vi "解析数据.vi"(8 "error in (no error)":errorcluster caption="错误输入（无错误）", 9 "当前模块数据属性":T1(array[cluster]), 10 "当前模块上一次的值":string[](array[string]), 11 "配置信息":string[](array[string])) -> (0 "error out":errorcluster caption="错误输出", 3 "输出数据":string)   [LabVIEW 2014]
doc: "该模板用于创建子VI。"
uses:
  glb/glb_data.vi
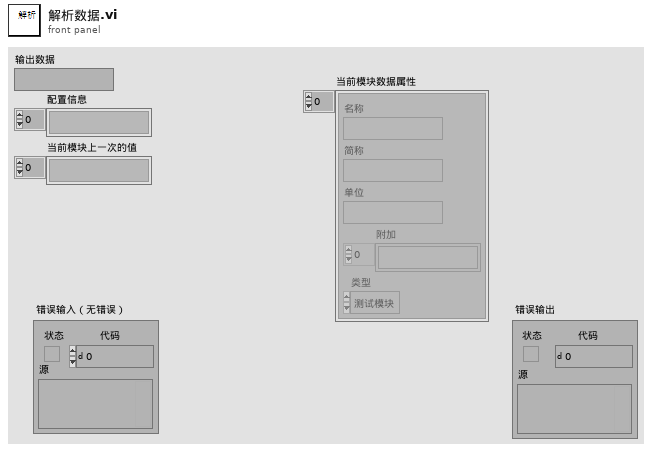
[diagram p1: front panel]
types:
  T1 = cluster{"名称":string, "简称":string, "单位":string, "附加":string[], "类型":enum16{"测试模块", "FPGA", "cRIO", "其他设备", "总体展示"}}[]
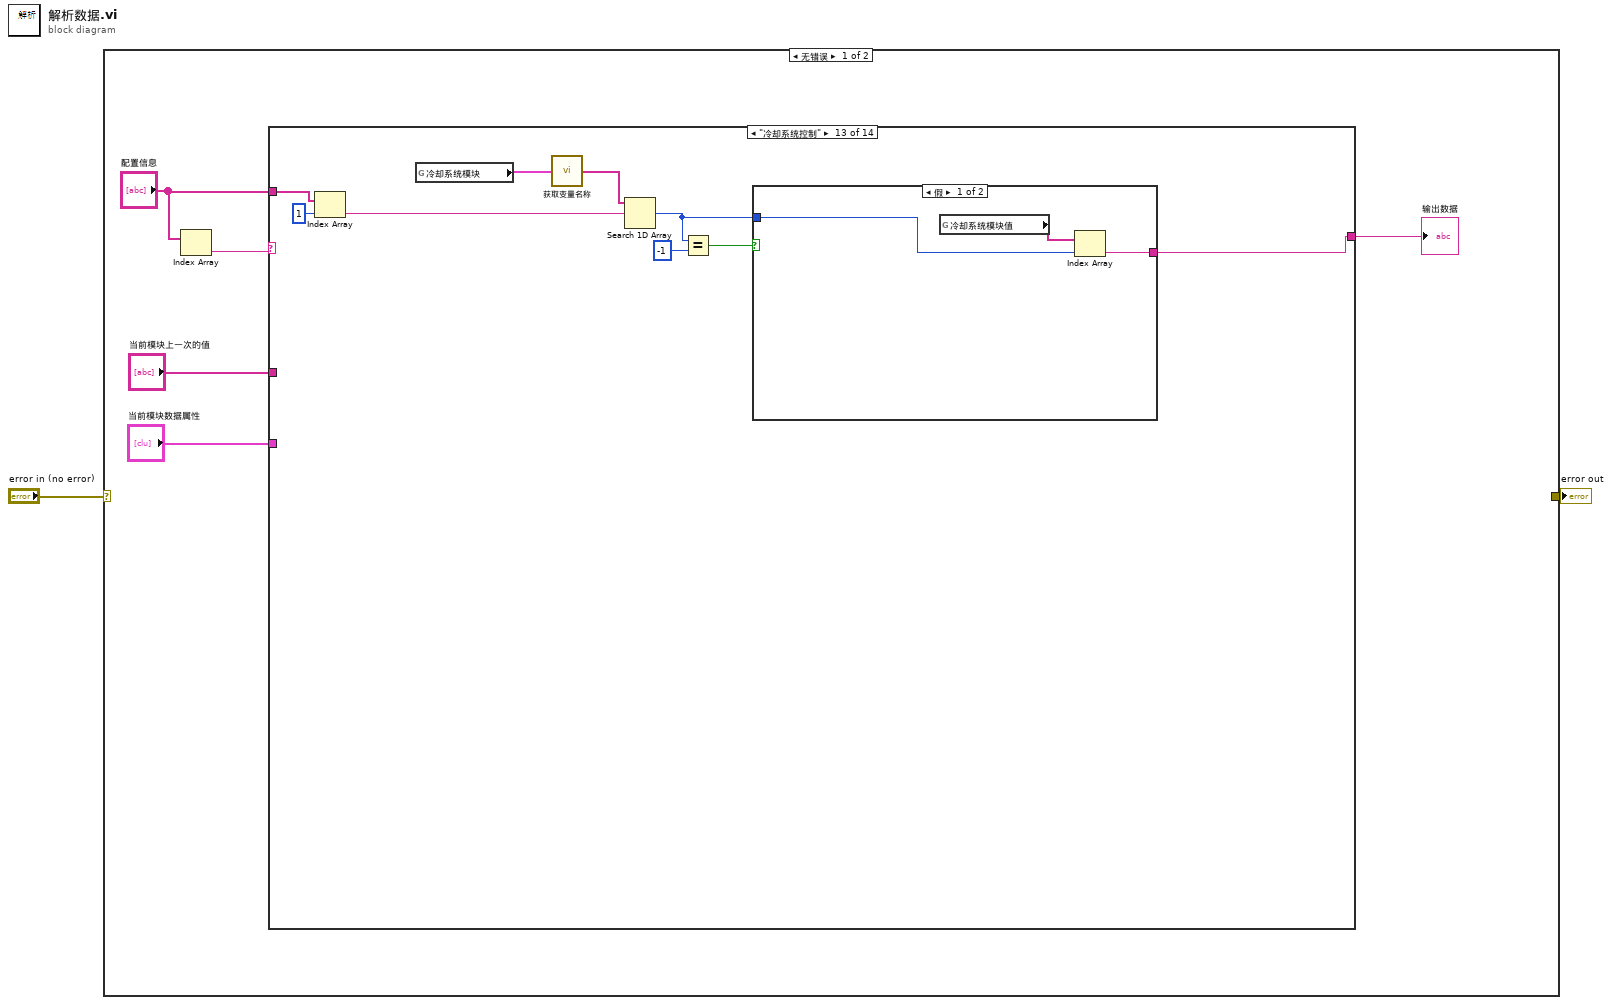
[diagram p0: block diagram]
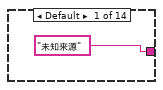
[diagram p2: hidden frame]
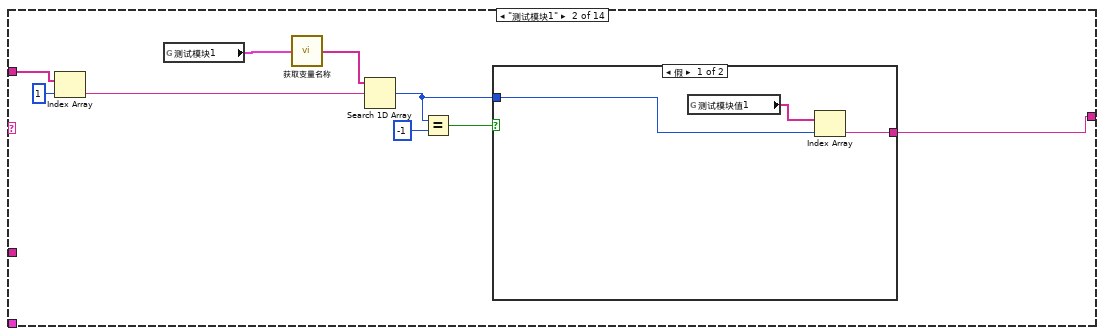
[diagram p3: hidden frame]
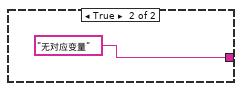
[diagram p4: hidden frame]
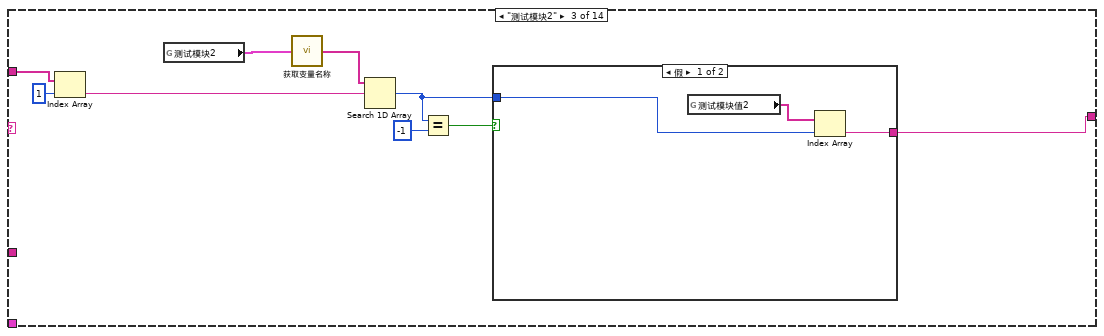
[diagram p5: hidden frame]
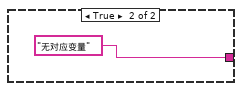
[diagram p6: hidden frame]
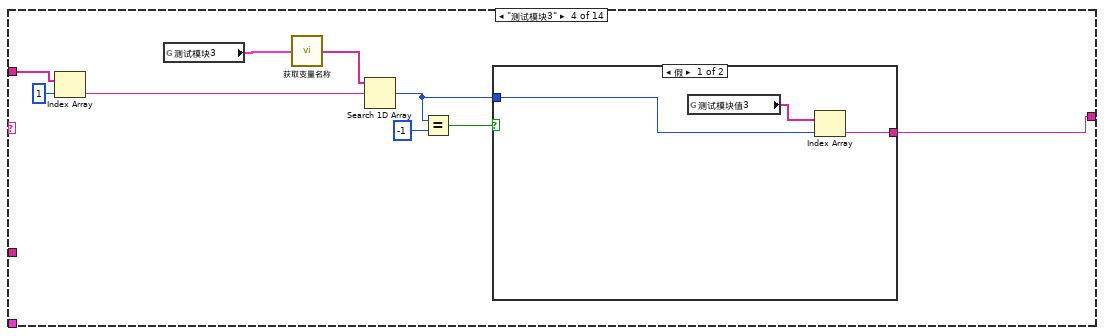
[diagram p7: hidden frame]
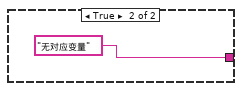
[diagram p8: hidden frame]
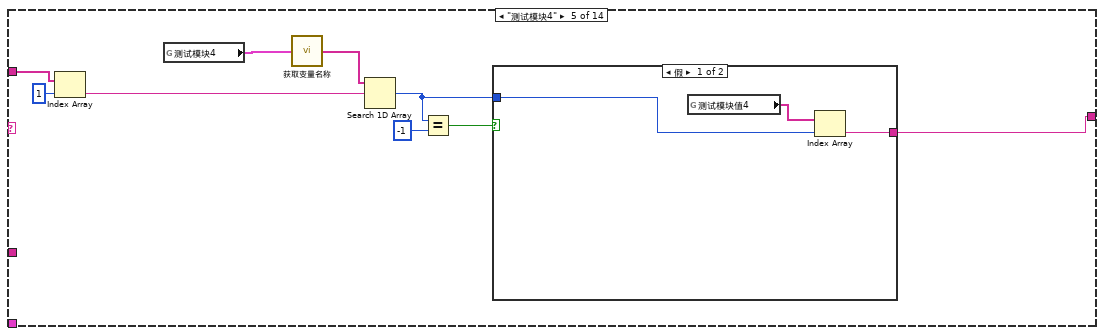
[diagram p9: hidden frame]
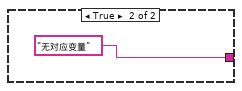
[diagram p10: hidden frame]
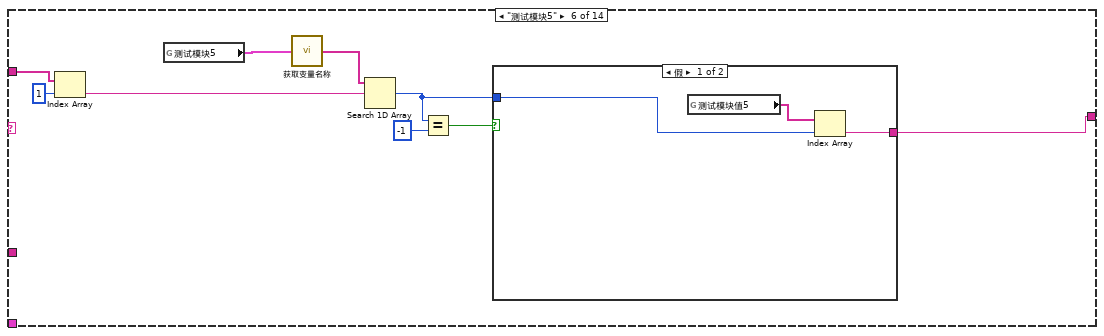
[diagram p11: hidden frame]
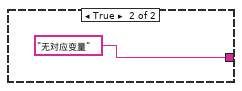
[diagram p12: hidden frame]
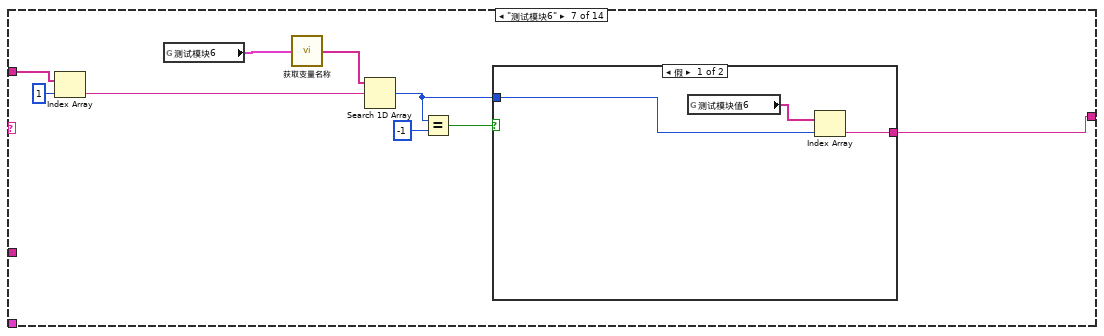
[diagram p13: hidden frame]
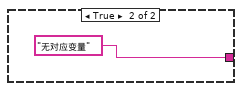
[diagram p14: hidden frame]
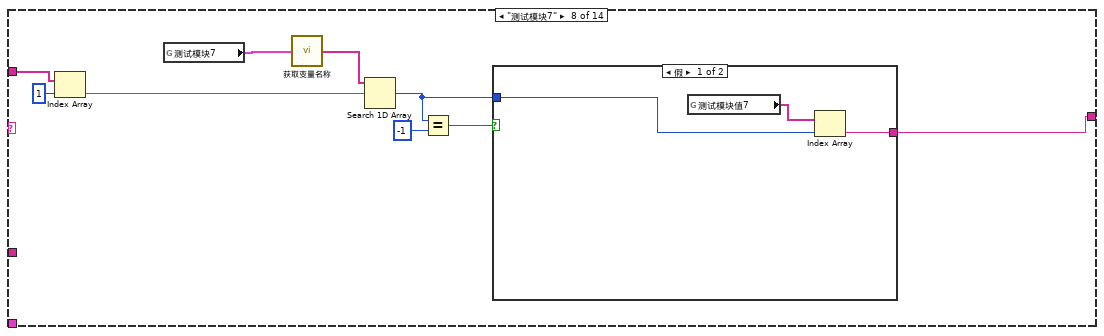
[diagram p15: hidden frame]
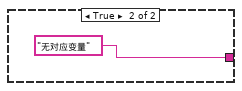
[diagram p16: hidden frame]
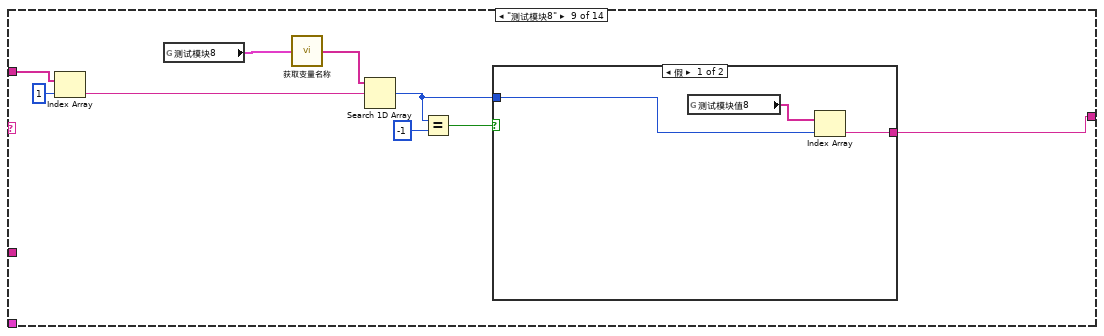
[diagram p17: hidden frame]
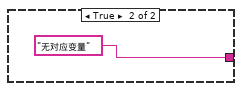
[diagram p18: hidden frame]
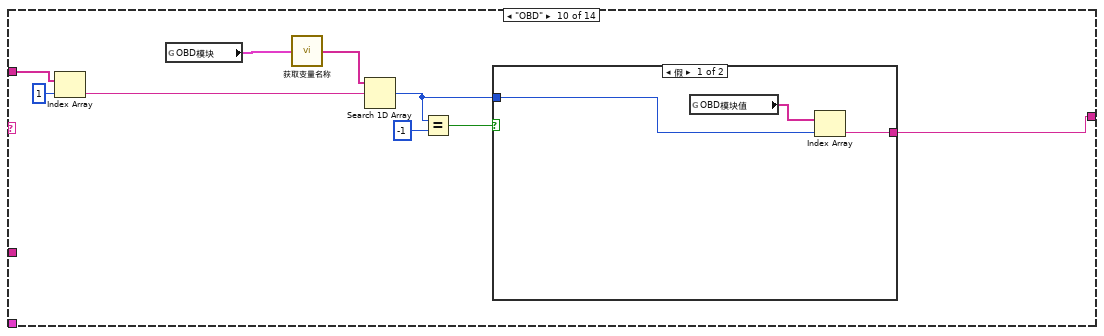
[diagram p19: hidden frame]
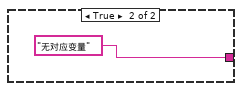
[diagram p20: hidden frame]
diagram:
  n1 = case shown="无错误" "error in (no error)" {
    selector: "error in (no error)" -> [_ w451]
    tunnel: [_ w451] -> w1
    frame No Error {
      n2 = Index Array(array="配置信息") -> (element=w6:string)  [unwired: 1 in]
      n3 = case shown="\"冷却系统控制\"" w6 {
        tunnel: ["未知来源" ("来源") w10 w23 w36 w49 w62 w75 w88 w101 w114 w127 w140 w153 w168] -> w7
        tunnel: "配置信息" -> [_ w17 w30 w43 w56 w69 w82 w95 w108 w121 w134 w147 w160 w167]
        tunnel: "当前模块上一次的值" -> [_ _ _ _ _ _ _ _ _ _ _ _ _ w165]
        tunnel: "当前模块数据属性" -> [_ _ _ _ _ _ _ _ _ _ _ _ _ w166]
        frame Default {
        }
        frame "测试模块1" {
          n4 = Index Array(array=w17, index=1 ("索引")) -> (element=w13:string)
          n5 = global read "glb_data.vi" "测试模块1"() -> (w15:T1)
          n6 = call "获取变量名称.vi"("属性数组"=w15) -> ("名称数组"=w14:string[])
          n7 = Search 1D Array(1D array=w14, element=w13) -> (index of element=w9:i32)  [unwired: 1 in]
          n8 = Equal?(x=w9, y=-1) -> (x = y?=w11:bool)
          n9 = case shown="假" w11 {
            tunnel: [w19 "无对应变量" ("来源")] -> w10
            tunnel: w9 -> [w18 _]
            frame False {
              n10 = global read "glb_data.vi" "测试模块值1"() -> (w20:string[])
              n11 = Index Array(array=w20, index=w18) -> (element=w19:string)
            }
            frame True {
            }
          }
        }
        frame "测试模块2" {
          n12 = Index Array(array=w30, index=1 ("索引")) -> (element=w26:string)
          n13 = global read "glb_data.vi" "测试模块2"() -> (w28:T1)
          n14 = call "获取变量名称.vi"("属性数组"=w28) -> ("名称数组"=w27:string[])
          n15 = Search 1D Array(1D array=w27, element=w26) -> (index of element=w22:i32)  [unwired: 1 in]
          n16 = Equal?(x=w22, y=-1) -> (x = y?=w24:bool)
          n17 = case shown="假" w24 {
            tunnel: [w32 "无对应变量" ("来源")] -> w23
            tunnel: w22 -> [w31 _]
            frame False {
              n18 = global read "glb_data.vi" "测试模块值2"() -> (w33:string[])
              n19 = Index Array(array=w33, index=w31) -> (element=w32:string)
            }
            frame True {
            }
          }
        }
        frame "测试模块3" {
          n20 = Index Array(array=w43, index=1 ("索引")) -> (element=w39:string)
          n21 = global read "glb_data.vi" "测试模块3"() -> (w41:T1)
          n22 = call "获取变量名称.vi"("属性数组"=w41) -> ("名称数组"=w40:string[])
          n23 = Search 1D Array(1D array=w40, element=w39) -> (index of element=w35:i32)  [unwired: 1 in]
          n24 = Equal?(x=w35, y=-1) -> (x = y?=w37:bool)
          n25 = case shown="假" w37 {
            tunnel: [w45 "无对应变量" ("来源")] -> w36
            tunnel: w35 -> [w44 _]
            frame False {
              n26 = global read "glb_data.vi" "测试模块值3"() -> (w46:string[])
              n27 = Index Array(array=w46, index=w44) -> (element=w45:string)
            }
            frame True {
            }
          }
        }
        frame "测试模块4" {
          n28 = Index Array(array=w56, index=1 ("索引")) -> (element=w52:string)
          n29 = global read "glb_data.vi" "测试模块4"() -> (w54:T1)
          n30 = call "获取变量名称.vi"("属性数组"=w54) -> ("名称数组"=w53:string[])
          n31 = Search 1D Array(1D array=w53, element=w52) -> (index of element=w48:i32)  [unwired: 1 in]
          n32 = Equal?(x=w48, y=-1) -> (x = y?=w50:bool)
          n33 = case shown="假" w50 {
            tunnel: [w58 "无对应变量" ("来源")] -> w49
            tunnel: w48 -> [w57 _]
            frame False {
              n34 = global read "glb_data.vi" "测试模块值4"() -> (w59:string[])
              n35 = Index Array(array=w59, index=w57) -> (element=w58:string)
            }
            frame True {
            }
          }
        }
        frame "测试模块5" {
          n36 = Index Array(array=w69, index=1 ("索引")) -> (element=w65:string)
          n37 = global read "glb_data.vi" "测试模块5"() -> (w67:T1)
          n38 = call "获取变量名称.vi"("属性数组"=w67) -> ("名称数组"=w66:string[])
          n39 = Search 1D Array(1D array=w66, element=w65) -> (index of element=w61:i32)  [unwired: 1 in]
          n40 = Equal?(x=w61, y=-1) -> (x = y?=w63:bool)
          n41 = case shown="假" w63 {
            tunnel: [w71 "无对应变量" ("来源")] -> w62
            tunnel: w61 -> [w70 _]
            frame False {
              n42 = global read "glb_data.vi" "测试模块值5"() -> (w72:string[])
              n43 = Index Array(array=w72, index=w70) -> (element=w71:string)
            }
            frame True {
            }
          }
        }
        frame "测试模块6" {
          n44 = Index Array(array=w82, index=1 ("索引")) -> (element=w78:string)
          n45 = global read "glb_data.vi" "测试模块6"() -> (w80:T1)
          n46 = call "获取变量名称.vi"("属性数组"=w80) -> ("名称数组"=w79:string[])
          n47 = Search 1D Array(1D array=w79, element=w78) -> (index of element=w74:i32)  [unwired: 1 in]
          n48 = Equal?(x=w74, y=-1) -> (x = y?=w76:bool)
          n49 = case shown="假" w76 {
            tunnel: [w84 "无对应变量" ("来源")] -> w75
            tunnel: w74 -> [w83 _]
            frame False {
              n50 = global read "glb_data.vi" "测试模块值6"() -> (w85:string[])
              n51 = Index Array(array=w85, index=w83) -> (element=w84:string)
            }
            frame True {
            }
          }
        }
        frame "测试模块7" {
          n52 = Index Array(array=w95, index=1 ("索引")) -> (element=w91:string)
          n53 = global read "glb_data.vi" "测试模块7"() -> (w93:T1)
          n54 = call "获取变量名称.vi"("属性数组"=w93) -> ("名称数组"=w92:string[])
          n55 = Search 1D Array(1D array=w92, element=w91) -> (index of element=w87:i32)  [unwired: 1 in]
          n56 = Equal?(x=w87, y=-1) -> (x = y?=w89:bool)
          n57 = case shown="假" w89 {
            tunnel: [w97 "无对应变量" ("来源")] -> w88
            tunnel: w87 -> [w96 _]
            frame False {
              n58 = global read "glb_data.vi" "测试模块值7"() -> (w98:string[])
              n59 = Index Array(array=w98, index=w96) -> (element=w97:string)
            }
            frame True {
            }
          }
        }
        frame "测试模块8" {
          n60 = Index Array(array=w108, index=1 ("索引")) -> (element=w104:string)
          n61 = global read "glb_data.vi" "测试模块8"() -> (w106:T1)
          n62 = call "获取变量名称.vi"("属性数组"=w106) -> ("名称数组"=w105:string[])
          n63 = Search 1D Array(1D array=w105, element=w104) -> (index of element=w100:i32)  [unwired: 1 in]
          n64 = Equal?(x=w100, y=-1) -> (x = y?=w102:bool)
          n65 = case shown="假" w102 {
            tunnel: [w110 "无对应变量" ("来源")] -> w101
            tunnel: w100 -> [w109 _]
            frame False {
              n66 = global read "glb_data.vi" "测试模块值8"() -> (w111:string[])
              n67 = Index Array(array=w111, index=w109) -> (element=w110:string)
            }
            frame True {
            }
          }
        }
        frame "OBD" {
          n68 = Index Array(array=w121, index=1 ("索引")) -> (element=w117:string)
          n69 = global read "glb_data.vi" "OBD模块"() -> (w119:T1)
          n70 = call "获取变量名称.vi"("属性数组"=w119) -> ("名称数组"=w118:string[])
          n71 = Search 1D Array(1D array=w118, element=w117) -> (index of element=w113:i32)  [unwired: 1 in]
          n72 = Equal?(x=w113, y=-1) -> (x = y?=w115:bool)
          n73 = case shown="假" w115 {
            tunnel: [w123 "无对应变量" ("来源")] -> w114
            tunnel: w113 -> [w122 _]
            frame False {
              n74 = global read "glb_data.vi" "OBD模块值"() -> (w124:string[])
              n75 = Index Array(array=w124, index=w122) -> (element=w123:string)
            }
            frame True {
            }
          }
        }
        frame "GPS" {
          n76 = Index Array(array=w134, index=1 ("索引")) -> (element=w130:string)
          n77 = global read "glb_data.vi" "GPS模块"() -> (w132:T1)
          n78 = call "获取变量名称.vi"("属性数组"=w132) -> ("名称数组"=w131:string[])
          n79 = Search 1D Array(1D array=w131, element=w130) -> (index of element=w126:i32)  [unwired: 1 in]
          n80 = Equal?(x=w126, y=-1) -> (x = y?=w128:bool)
          n81 = case shown="假" w128 {
            tunnel: [w136 "无对应变量" ("来源")] -> w127
            tunnel: w126 -> [w135 _]
            frame False {
              n82 = global read "glb_data.vi" "GPS模块值"() -> (w137:string[])
              n83 = Index Array(array=w137, index=w135) -> (element=w136:string)
            }
            frame True {
            }
          }
        }
        frame "cRIO" {
          n84 = Index Array(array=w147, index=1 ("索引")) -> (element=w143:string)
          n85 = global read "glb_data.vi" "cRIO模块"() -> (w145:T1)
          n86 = call "获取变量名称.vi"("属性数组"=w145) -> ("名称数组"=w144:string[])
          n87 = Search 1D Array(1D array=w144, element=w143) -> (index of element=w139:i32)  [unwired: 1 in]
          n88 = Equal?(x=w139, y=-1) -> (x = y?=w141:bool)
          n89 = case shown="假" w141 {
            tunnel: [w149 "无对应变量" ("来源")] -> w140
            tunnel: w139 -> [w148 _]
            frame False {
              n90 = global read "glb_data.vi" "cRIO模块值"() -> (w150:string[])
              n91 = Index Array(array=w150, index=w148) -> (element=w149:string)
            }
            frame True {
            }
          }
        }
        frame "冷却系统控制" {
          n92 = Index Array(array=w160, index=1 ("索引")) -> (element=w156:string)
          n93 = global read "glb_data.vi" "冷却系统模块"() -> (w158:T1)
          n94 = call "获取变量名称.vi"("属性数组"=w158) -> ("名称数组"=w157:string[])
          n95 = Search 1D Array(1D array=w157, element=w156) -> (index of element=w152:i32)  [unwired: 1 in]
          n96 = Equal?(x=w152, y=-1) -> (x = y?=w154:bool)
          n97 = case shown="假" w154 {
            tunnel: [w162 "无对应变量" ("来源")] -> w153
            tunnel: w152 -> [w161 _]
            frame False {
              n98 = global read "glb_data.vi" "冷却系统模块值"() -> (w163:string[])
              n99 = Index Array(array=w163, index=w161) -> (element=w162:string)
            }
            frame True {
            }
          }
        }
        frame "运算" {
          n100 = Index Array(array=w167, index=1 ("索引")) -> (element=w169:string)
          n101 = case shown="\"散热量计算\"" w169 {
            tunnel: ["未定义运算方法" w172 w178 w212 w246 w280 w314 w339 w368 w411] -> w168
            tunnel: w167 -> [_ w174 w189 w223 w257 w291 w321 w345 w374 w416]
            tunnel: w166 -> [_ _ w187 w221 w255 w289 w319 w343 w372 w414]
            tunnel: w165 -> [_ _ w177 w211 w245 w279 w313 w338 w367 w410]
            frame Default {
            }
            frame "常数" {
              n102 = Index Array(array=w174, index=2 ("索引")) -> (element=w172:string)
            }
            frame "加" {
              n103 = Index Array(array=w189, index #1=2 ("索引")) -> (element #1=w180:string, element #2=w179:string)  [unwired: 1 in]
              n104 = call "获取变量名称.vi"("属性数组"=w187) -> ("名称数组"=w186:string[])
              n105 = Search 1D Array(1D array=w186, element=w180) -> (index of element=w176:i32)  [unwired: 1 in]
              n106 = Search 1D Array(1D array=w186, element=w179) -> (index of element=w175:i32)  [unwired: 1 in]
              n107 = Equal?(x=w176, y=-1) -> (x = y?=w182:bool)
              n108 = Equal?(x=w175, y=-1) -> (x = y?=w181:bool)
              n109 = Or(x=w182, y=w181) -> (x .or. y?=w183:bool)
              n110 = case shown="假" w183 {
                tunnel: w182 -> [_ w208]
                tunnel: w181 -> [_ w207]
                tunnel: w180 -> [_ w206]
                tunnel: w179 -> [_ w203]
                tunnel: [w190 w199] -> w178
                tunnel: w177 -> [w197 _]
                tunnel: w176 -> [w198 _]
                tunnel: w175 -> [w196 _]
                frame False {
                  n111 = Index Array(array=w197, index=w198) -> (element=w195:string)
                  n112 = Index Array(array=w197, index=w196) -> (element=w194:string)
                  n113 = Fract/Exp String To Number(string=w195) -> (number=w193:dbl)  [unwired: 3 in, 1 out]
                  n114 = Fract/Exp String To Number(string=w194) -> (number=w192:dbl)  [unwired: 3 in, 1 out]
                  n115 = Add(x=w193, y=w192) -> (x+y=w191:dbl)
                  n116 = Number To Exponential String(number=w191) -> (E-format string=w190:string)  [unwired: 3 in]
                }
                frame True {
                  n117 = Select(t=w203, s=w207, f="") -> (s? t:f=w200:string)
                  n118 = Select(t=w206, s=w208, f="") -> (s? t:f=w201:string)
                  n119 = Concatenate Strings("运算，未找到", w201, w200) -> (w199:string)
                }
              }
            }
            frame "减" {
              n120 = Index Array(array=w223, index #1=2 ("索引")) -> (element #1=w214:string, element #2=w213:string)  [unwired: 1 in]
              n121 = call "获取变量名称.vi"("属性数组"=w221) -> ("名称数组"=w220:string[])
              n122 = Search 1D Array(1D array=w220, element=w214) -> (index of element=w210:i32)  [unwired: 1 in]
              n123 = Search 1D Array(1D array=w220, element=w213) -> (index of element=w209:i32)  [unwired: 1 in]
              n124 = Equal?(x=w210, y=-1) -> (x = y?=w216:bool)
              n125 = Equal?(x=w209, y=-1) -> (x = y?=w215:bool)
              n126 = Or(x=w216, y=w215) -> (x .or. y?=w217:bool)
              n127 = case shown="假" w217 {
                tunnel: w216 -> [_ w242]
                tunnel: w215 -> [_ w241]
                tunnel: w214 -> [_ w240]
                tunnel: w213 -> [_ w237]
                tunnel: [w224 w233] -> w212
                tunnel: w211 -> [w231 _]
                tunnel: w210 -> [w232 _]
                tunnel: w209 -> [w230 _]
                frame False {
                  n128 = Index Array(array=w231, index=w232) -> (element=w229:string)
                  n129 = Index Array(array=w231, index=w230) -> (element=w228:string)
                  n130 = Fract/Exp String To Number(string=w229) -> (number=w227:dbl)  [unwired: 3 in, 1 out]
                  n131 = Fract/Exp String To Number(string=w228) -> (number=w226:dbl)  [unwired: 3 in, 1 out]
                  n132 = Subtract(x=w227, y=w226) -> (x-y=w225:dbl)
                  n133 = Number To Exponential String(number=w225) -> (E-format string=w224:string)  [unwired: 3 in]
                }
                frame True {
                  n134 = Select(t=w237, s=w241, f="") -> (s? t:f=w234:string)
                  n135 = Select(t=w240, s=w242, f="") -> (s? t:f=w235:string)
                  n136 = Concatenate Strings("运算，未找到", w235, w234) -> (w233:string)
                }
              }
            }
            frame "乘" {
              n137 = Index Array(array=w257, index #1=2 ("索引")) -> (element #1=w248:string, element #2=w247:string)  [unwired: 1 in]
              n138 = call "获取变量名称.vi"("属性数组"=w255) -> ("名称数组"=w254:string[])
              n139 = Search 1D Array(1D array=w254, element=w248) -> (index of element=w244:i32)  [unwired: 1 in]
              n140 = Search 1D Array(1D array=w254, element=w247) -> (index of element=w243:i32)  [unwired: 1 in]
              n141 = Equal?(x=w244, y=-1) -> (x = y?=w250:bool)
              n142 = Equal?(x=w243, y=-1) -> (x = y?=w249:bool)
              n143 = Or(x=w250, y=w249) -> (x .or. y?=w251:bool)
              n144 = case shown="假" w251 {
                tunnel: w250 -> [_ w276]
                tunnel: w249 -> [_ w275]
                tunnel: w248 -> [_ w274]
                tunnel: w247 -> [_ w271]
                tunnel: [w258 w267] -> w246
                tunnel: w245 -> [w265 _]
                tunnel: w244 -> [w266 _]
                tunnel: w243 -> [w264 _]
                frame False {
                  n145 = Index Array(array=w265, index=w266) -> (element=w263:string)
                  n146 = Index Array(array=w265, index=w264) -> (element=w262:string)
                  n147 = Fract/Exp String To Number(string=w263) -> (number=w261:dbl)  [unwired: 3 in, 1 out]
                  n148 = Fract/Exp String To Number(string=w262) -> (number=w260:dbl)  [unwired: 3 in, 1 out]
                  n149 = Multiply(x=w261, y=w260) -> (x*y=w259:dbl)
                  n150 = Number To Exponential String(number=w259) -> (E-format string=w258:string)  [unwired: 3 in]
                }
                frame True {
                  n151 = Select(t=w271, s=w275, f="") -> (s? t:f=w268:string)
                  n152 = Select(t=w274, s=w276, f="") -> (s? t:f=w269:string)
                  n153 = Concatenate Strings("运算，未找到", w269, w268) -> (w267:string)
                }
              }
            }
            frame "除" {
              n154 = Index Array(array=w291, index #1=2 ("索引")) -> (element #1=w282:string, element #2=w281:string)  [unwired: 1 in]
              n155 = call "获取变量名称.vi"("属性数组"=w289) -> ("名称数组"=w288:string[])
              n156 = Search 1D Array(1D array=w288, element=w282) -> (index of element=w278:i32)  [unwired: 1 in]
              n157 = Search 1D Array(1D array=w288, element=w281) -> (index of element=w277:i32)  [unwired: 1 in]
              n158 = Equal?(x=w278, y=-1) -> (x = y?=w284:bool)
              n159 = Equal?(x=w277, y=-1) -> (x = y?=w283:bool)
              n160 = Or(x=w284, y=w283) -> (x .or. y?=w285:bool)
              n161 = case shown="假" w285 {
                tunnel: w284 -> [_ w310]
                tunnel: w283 -> [_ w309]
                tunnel: w282 -> [_ w308]
                tunnel: w281 -> [_ w305]
                tunnel: [w292 w301] -> w280
                tunnel: w279 -> [w299 _]
                tunnel: w278 -> [w300 _]
                tunnel: w277 -> [w298 _]
                frame False {
                  n162 = Index Array(array=w299, index=w300) -> (element=w297:string)
                  n163 = Index Array(array=w299, index=w298) -> (element=w296:string)
                  n164 = Fract/Exp String To Number(string=w297) -> (number=w295:dbl)  [unwired: 3 in, 1 out]
                  n165 = Fract/Exp String To Number(string=w296) -> (number=w294:dbl)  [unwired: 3 in, 1 out]
                  n166 = Divide(x=w295, y=w294) -> (x/y=w293:dbl)
                  n167 = Number To Exponential String(number=w293) -> (E-format string=w292:string)  [unwired: 3 in]
                }
                frame True {
                  n168 = Select(t=w305, s=w309, f="") -> (s? t:f=w302:string)
                  n169 = Select(t=w308, s=w310, f="") -> (s? t:f=w303:string)
                  n170 = Concatenate Strings("运算，未找到", w303, w302) -> (w301:string)
                }
              }
            }
            frame "幂运算" {
              n171 = Index Array(array=w321, index #1=2 ("索引")) -> (element #1=w316:string, element #2=w315:string)  [unwired: 1 in]
              n172 = call "获取变量名称.vi"("属性数组"=w319) -> ("名称数组"=w318:string[])
              n173 = Search 1D Array(1D array=w318, element=w316) -> (index of element=w312:i32)  [unwired: 1 in]
              n174 = Equal?(x=w312, y=-1) -> (x = y?=w311:bool)
              n175 = case shown="假" w311 {
                tunnel: w311 -> [_ w335]
                tunnel: w316 -> [_ w334]
                tunnel: w315 -> [w325 _]
                tunnel: [w326 w330] -> w314
                tunnel: w313 -> [w328 _]
                tunnel: w312 -> [w329 _]
                frame False {
                  n176 = Index Array(array=w328, index=w329) -> (element=w327:string)
                  n177 = Fract/Exp String To Number(string=w327) -> (number=w323:dbl)  [unwired: 3 in, 1 out]
                  n178 = Fract/Exp String To Number(string=w325) -> (number=w324:dbl)  [unwired: 3 in, 1 out]
                  n179 = Power Of X(1:w323, 2:w324) -> (0:w322:dbl)
                  n180 = Number To Exponential String(number=w322) -> (E-format string=w326:string)  [unwired: 3 in]
                }
                frame True {
                  n181 = Select(t=w334, s=w335, f="") -> (s? t:f=w331:string)
                  n182 = Concatenate Strings("运算，未找到", w331) -> (w330:string)
                }
              }
            }
            frame "微分" {
              n183 = Index Array(array=w345, index=2 ("索引")) -> (element=w340:string)
              n184 = call "获取变量名称.vi"("属性数组"=w343) -> ("名称数组"=w342:string[])
              n185 = Search 1D Array(1D array=w342, element=w340) -> (index of element=w337:i32)  [unwired: 1 in]
              n186 = Equal?(x=w337, y=-1) -> (x = y?=w336:bool)
              n187 = case shown="假" w336 {
                tunnel: w336 -> [_ w364]
                tunnel: w340 -> [_ w363]
                tunnel: [w354 w359] -> w339
                tunnel: w338 -> [w357 _]
                tunnel: w337 -> [w358 _]
                frame False {
                  n188 = Tick Count (ms)() -> (millisecond timer value=w352:u32)
                  n189 = feedback #1() -> (w351:u32)  [unwired: 1 in]
                  n190 = feedback-in #1(w352) -> ()
                  n191 = Index Array(array=w357, index=w358) -> (element=w356:string)
                  n192 = Subtract(x=w352, y=w351) -> (x-y=w350:u32)
                  n193 = feedback #2() -> (w346:dbl)  [unwired: 1 in]
                  n194 = Fract/Exp String To Number(string=w356) -> (number=w347:dbl)  [unwired: 3 in, 1 out]
                  n195 = feedback-in #2(w347) -> ()
                  n196 = Divide(x=w350, y=u32 1000) -> (x/y=w348:dbl)
                  n197 = Subtract(x=w347, y=w346) -> (x-y=w353:dbl)
                  n198 = Divide(x=w353, y=w348) -> (x/y=w355:dbl)
                  n199 = Number To Exponential String(number=w355) -> (E-format string=w354:string)  [unwired: 3 in]
                }
                frame True {
                  (unwired) ""
                  n200 = Select(t=w363, s=w364, f="") -> (s? t:f=w360:string)
                  n201 = Concatenate Strings("运算，未找到", w360) -> (w359:string)
                }
              }
            }
            frame "积分" {
              n202 = Index Array(array=w374, index=2 ("索引")) -> (element=w369:string)
              n203 = call "获取变量名称.vi"("属性数组"=w372) -> ("名称数组"=w371:string[])
              n204 = Search 1D Array(1D array=w371, element=w369) -> (index of element=w366:i32)  [unwired: 1 in]
              n205 = Equal?(x=w366, y=-1) -> (x = y?=w365:bool)
              n206 = case shown="假" w365 {
                tunnel: w365 -> [_ w393]
                tunnel: w369 -> [_ w392]
                tunnel: [w384 w388] -> w368
                tunnel: w367 -> [w386 _]
                tunnel: w366 -> [w387 _]
                frame False {
                  n207 = Tick Count (ms)() -> (millisecond timer value=w383:u32)
                  n208 = feedback #3() -> (w382:u32)  [unwired: 1 in]
                  n209 = feedback-in #3(w383) -> ()
                  n210 = Index Array(array=w386, index=w387) -> (element=w385:string)
                  n211 = Subtract(x=w383, y=w382) -> (x-y=w381:u32)
                  n212 = Fract/Exp String To Number(string=w385) -> (number=w378:dbl)  [unwired: 3 in, 1 out]
                  n213 = Divide(x=w381, y=u32 1000) -> (x/y=w379:dbl)
                  n214 = Multiply(x=w378, y=w379) -> (x*y=w377:dbl)
                  n215 = feedback #4() -> (w376:dbl)  [unwired: 1 in]
                  n216 = Add(x=w376, y=w377) -> (x+y=w375:dbl)
                  n217 = feedback-in #4(w375) -> ()
                  n218 = Number To Exponential String(number=w375) -> (E-format string=w384:string)  [unwired: 3 in]
                }
                frame True {
                  (unwired) ""
                  n219 = Select(t=w392, s=w393, f="") -> (s? t:f=w389:string)
                  n220 = Concatenate Strings("运算，未找到", w389) -> (w388:string)
                }
              }
            }
            frame "散热量计算" {
              n221 = Index Array(array=w416, index #1=2 ("索引")) -> (element #1=w412:string, element #2=w399:string, element #3=w398:string, element #4=w397:string)  [unwired: 3 in]
              n222 = call "获取变量名称.vi"("属性数组"=w414) -> ("名称数组"=w405:string[])
              n223 = Search 1D Array(1D array=w405, element=w412) -> (index of element=w409:i32)  [unwired: 1 in]
              n224 = Search 1D Array(1D array=w405, element=w399) -> (index of element=w396:i32)  [unwired: 1 in]
              n225 = Search 1D Array(1D array=w405, element=w398) -> (index of element=w395:i32)  [unwired: 1 in]
              n226 = Search 1D Array(1D array=w405, element=w397) -> (index of element=w394:i32)  [unwired: 1 in]
              n227 = Equal?(x=w409, y=-1) -> (x = y?=w404:bool)
              n228 = Equal?(x=w396, y=-1) -> (x = y?=w402:bool)
              n229 = Equal?(x=w395, y=-1) -> (x = y?=w401:bool)
              n230 = Equal?(x=w394, y=-1) -> (x = y?=w400:bool)
              n231 = Compound Arithmetic op=OR(w404, w402, w401, w400) -> (w403:bool)
              n232 = case shown="假" w403 {
                tunnel: w404 -> [_ w450]
                tunnel: w412 -> [_ w449]
                tunnel: [w430 w445] -> w411
                tunnel: w410 -> [w426 _]
                tunnel: w409 -> [w432 _]
                tunnel: w402 -> [_ w441]
                tunnel: w401 -> [_ w440]
                tunnel: w400 -> [_ w439]
                tunnel: w399 -> [_ w438]
                tunnel: w398 -> [_ w437]
                tunnel: w397 -> [_ w436]
                tunnel: w396 -> [w419 _]
                tunnel: w395 -> [w418 _]
                tunnel: w394 -> [w417 _]
                frame False {
                  n233 = Index Array(array=w426, index=w432) -> (element=w431:string)
                  n234 = Index Array(array=w426, index=w419) -> (element=w429:string)
                  n235 = Index Array(array=w426, index=w418) -> (element=w428:string)
                  n236 = Index Array(array=w426, index=w417) -> (element=w427:string)
                  n237 = Fract/Exp String To Number(string=w431) -> (number=w423:dbl)  [unwired: 3 in, 1 out]
                  n238 = Fract/Exp String To Number(string=w429) -> (number=w422:dbl)  [unwired: 3 in, 1 out]
                  n239 = Fract/Exp String To Number(string=w428) -> (number=w425:dbl)  [unwired: 3 in, 1 out]
                  n240 = Fract/Exp String To Number(string=w427) -> (number=w424:dbl)  [unwired: 3 in, 1 out]
                  n241 = Subtract(x=w425, y=w424) -> (x-y=w421:dbl)
                  n242 = Compound Arithmetic op=MULTIPLY(w423, w422, w421) -> (w420:dbl)
                  n243 = Number To Exponential String(number=w420) -> (E-format string=w430:string)  [unwired: 3 in]
                }
                frame True {
                  n244 = Select(t=w449, s=w450, f="") -> (s? t:f=w446:string)
                  n245 = Select(t=w438, s=w441, f="") -> (s? t:f=w435:string)
                  n246 = Select(t=w436, s=w439, f="") -> (s? t:f=w433:string)
                  n247 = Select(t=w437, s=w440, f="") -> (s? t:f=w434:string)
                  n248 = Concatenate Strings("运算，未找到", w446, w435, w434, w433) -> (w445:string)
                }
              }
            }
          }
        }
      }
      "输出数据" <- w7
    }
    frame Error {
    }
  }
  "error out" <- w1
